vi "SetpointAndPastR.vi"(9 "Horizon":i32, 10 "Numeric":i32, 11 "dt (ms)":u32) -> (2 "Future_R":T1, 3 "b":dbl)   [LabVIEW 2016]
uses:
  <vilib>/Analysis/Matrix/Datatypes/RealMatrix.ctl
  <vilib>/Analysis/Matrix/Numeric/Conversions/Array To Matrix - RA.vi
  <vilib>/Analysis/Matrix/NI_Matrix.lvlib
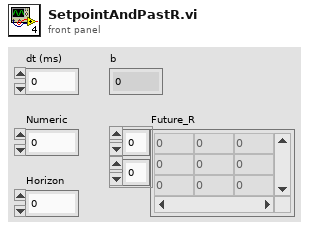
[diagram p1: front panel]
types:
  T1 = typedef "NI_Matrix.lvlib/RealMatrix.ctl" = dbl[][]
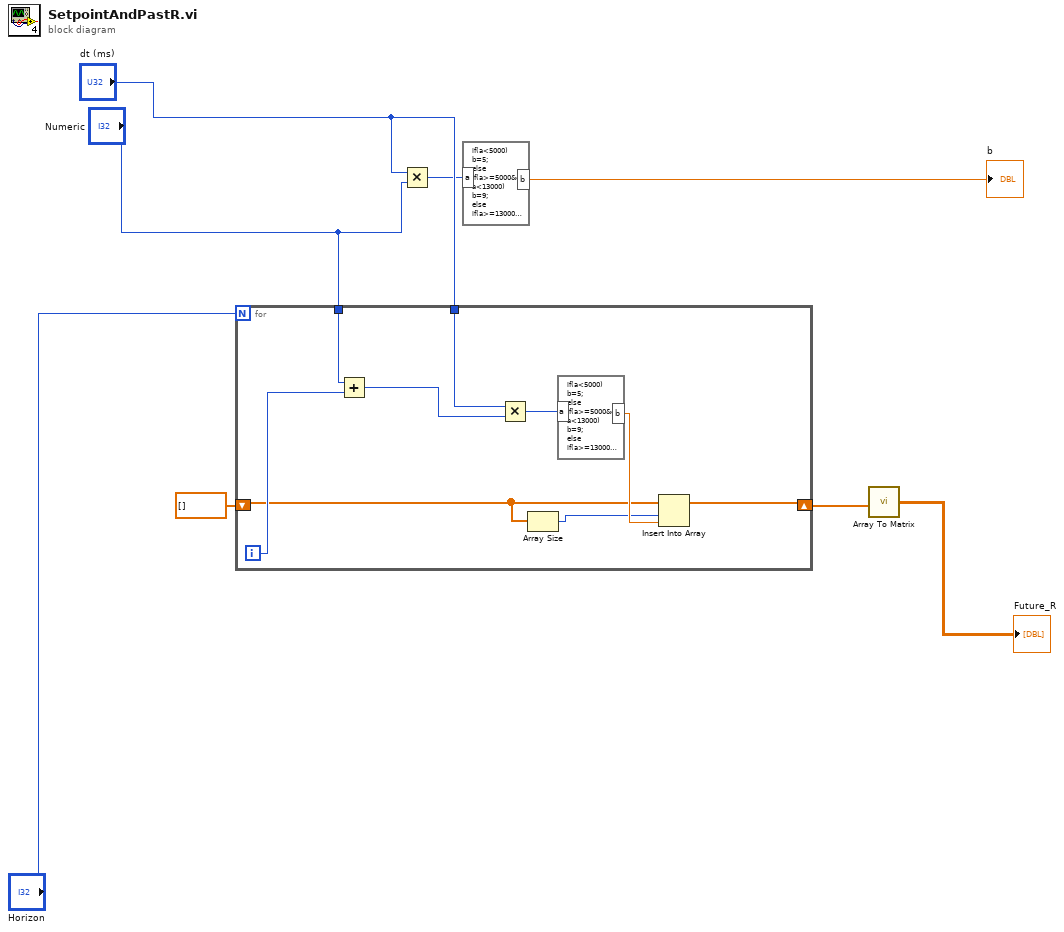
[diagram p0: block diagram]
diagram:
  n1 = for {
    N: "Horizon" -> [_]
    tunnel: "Numeric" -> [w17]
    tunnel: "dt (ms)" -> [w14]
    shift-right: [w11] -> w5
    shift-left: dbl[] [] -> [w10]
    i -> [w16]
    n2 = Add(x=w17, y=w16) -> (x+y=w15:i32)
    n3 = Multiply(x=w14, y=w15) -> (x*y=w13:u32)
    n4 = Array Size(array=w10) -> (size(s)=w9:i32)
    n5 = formula code="if(a<5000)\nb=5;\nelse \nif(a>=5000&&a<13000)\nb=9;\nelse\nif(a>=13000&&a<18000)\nb=13;\nelse\nif(a>=18000&&a<23000)\nb=7;\nelse\nif(a>=23000&&a<33000)\nb=-8;\nelse\nif(a>=33000)\nb=0;"("a"=w13) -> ("b"=w12:dbl)
    n6 = Insert Into Array(array=w10, index=w9, new element=w12) -> (w11:dbl[])
  }
  n7 = Multiply(x="dt (ms)", y="Numeric") -> (x*y=w1:u32)
  n8 = formula code="if(a<5000)\nb=5;\nelse \nif(a>=5000&&a<13000)\nb=9;\nelse\nif(a>=13000&&a<18000)\nb=13;\nelse\nif(a>=18000&&a<23000)\nb=7;\nelse\nif(a>=23000&&a<33000)\nb=-8;\nelse\nif(a>=33000)\nb=0;"("a"=w1) -> ("b"=→"b":dbl)
  n9 = call-poly <vilib>:"Array To Matrix.vi"("Real 1D Array"=w5) -> ("Real Matrix (Column Vector)"=→"Future_R":T1)
